vi "Resize Message String & 3-button Dialog Window.vi"(6 "Max Number of Lines":i32, 8 "Error In":errorcluster, 9 "Message":string, 10 "output Controls & Indicators":T1, 11 "VI Refnum":refnum<vi>) -> (0 "Error Out":errorcluster, 3 "VI Refnum out":refnum<vi>)   [LabVIEW 2021, in "GUI.lvlib"]
uses:
  GUI.lvlib
  Error/Error.lvlib
  Buttons/Buttons.lvlib
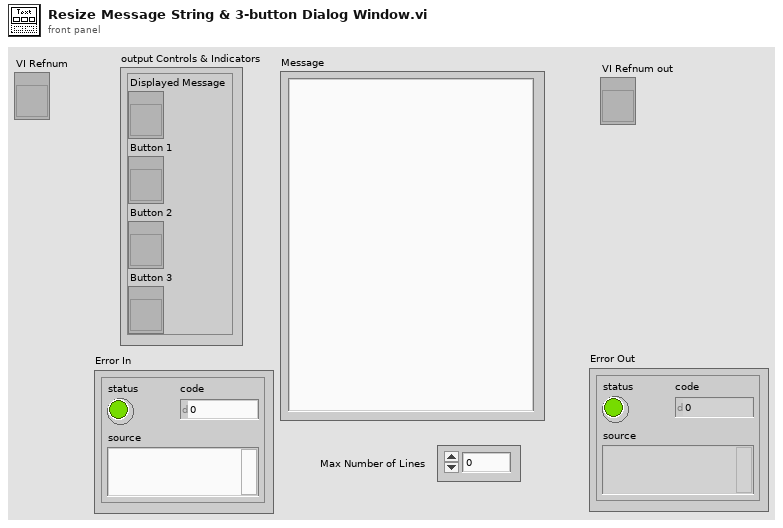
[diagram p1: front panel]
types:
  T1 = cluster{"Displayed Message":refnum<vi>, "Button 1":refnum<vi>, "Button 2":refnum<vi>, "Button 3":refnum<vi>}
  T2 = typedef "LVRectTypeDef.ctl" = cluster{"Left":i16, "Top":i16, "Right":i16, "Bottom":i16}
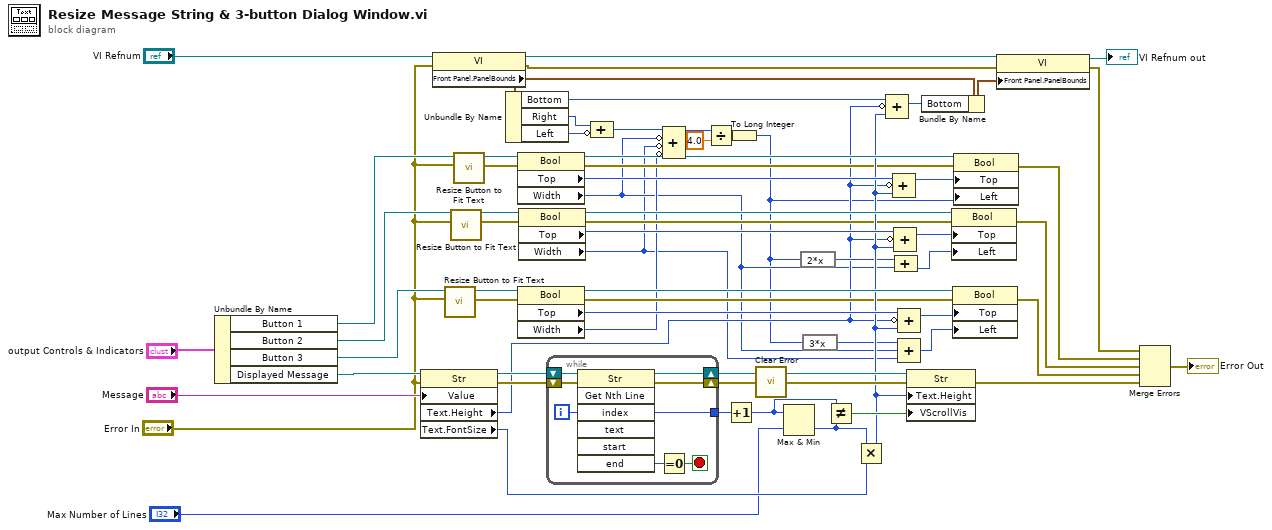
[diagram p0: block diagram]
diagram:
  n1 = Unbundle By Name("output Controls & Indicators") -> ("Button 1"=w13:refnum<vi>, "Button 2"=w21:refnum<vi>, "Button 3"=w41:refnum<vi>, "Displayed Message"=w51:refnum<vi>)
  n2 = property class="Str"(reference=w51, error in="Error In", "Value"="Message") -> (reference out=w65:refnum<vi>, error out=w64:errorcluster, "Text.Height"=w4:u32, "Text.FontSize"=w61:u32)
  n3 = property class="VI"(reference="VI Refnum", error in="Error In") -> (reference out=w47:refnum<vi>, error out=w46:errorcluster, "Front Panel.PanelBounds"=w49:T2)
  n4 = call "Resize Button to Fit Text.vi"("error in (no error)"="Error In", "Boolean in"=w41) -> ("error out"=w22:errorcluster, "Boolean out"=w23:refnum<vi>)  [unwired: 8 in]
  n5 = call "Resize Button to Fit Text.vi"("error in (no error)"="Error In", "Boolean in"=w21) -> ("error out"=w19:errorcluster, "Boolean out"=w20:refnum<vi>)  [unwired: 8 in]
  n6 = call "Resize Button to Fit Text.vi"("error in (no error)"="Error In", "Boolean in"=w13) -> ("error out"=w10:errorcluster, "Boolean out"=w12:refnum<vi>)  [unwired: 8 in]
  n7 = Unbundle By Name(w49) -> ("Bottom"=w50:i16, "Right"=w8:i16, "Left"=w26:i16)
  n8 = property class="Bool"(reference=w12, error in=w10) -> (reference out=w43:refnum<vi>, error out=w32:errorcluster, "Top"=w44:i32, "Width"=w3:u32)
  n9 = property class="Bool"(reference=w23, error in=w22) -> (reference out=w39:refnum<vi>, error out=w30:errorcluster, "Top"=w36:i32, "Width"=w27:u32)
  n10 = property class="Bool"(reference=w20, error in=w19) -> (reference out=w40:refnum<vi>, error out=w31:errorcluster, "Top"=w38:i32, "Width"=w2:u32)
  n11 = while {
    shift-right: [w71] -> w59
    shift-left: w64 -> [w72]
    shift-right: [w70] -> w60
    shift-left: w65 -> [w73]
    tunnel: [w68] -> w62
    i -> [w68]
    stop <- w67 stop-if-true
    n12 = invoke class="Str" method="Get Nth Line"(reference=w73, error in=w72, "index"=w68) -> (reference out=w70:refnum<vi>, error out=w71:errorcluster, "end"=w69:u32)  [unwired: 4 in, 4 out]
    n13 = Equal To 0?(x=w69) -> (x = 0?=w67:bool)
  }
  n14 = Compound Arithmetic op=ADD(w8, invert w26) -> (w25:i16)
  n15 = Compound Arithmetic op=ADD(w25, invert w3, invert w2, invert w27) -> (w29:u32)
  n16 = Divide(x=w29, y=4.0) -> (x/y=w6:dbl)
  n17 = Increment(x=w62) -> (x+1=w55:i32)
  n18 = To Long Integer(number=w6) -> (32bit integer=w1:i32)
  n19 = call "Clear Error.vi"("Error In"=w59) -> ("no Error Out"=w57:errorcluster)  [unwired: 8 in]
  n20 = Max & Min(x=w55, y="Max Number of Lines") -> (min(x,y)=w56:i32)  [unwired: 1 out]
  n21 = expression code="2*x"(w1) -> (w7:i32)
  n22 = expression code="3*x"(w1) -> (w5:i32)
  n23 = Not Equal?(x=w55, y=w56) -> (x != y?=w54:bool)
  n24 = Multiply(x=w56, y=w61) -> (x*y=w35:u32)
  n25 = Compound Arithmetic op=ADD(w50, invert w4, w35) -> (w48:u32)
  n26 = Compound Arithmetic op=ADD(w44, invert w4, w35) -> (w42:u32)
  n27 = Compound Arithmetic op=ADD(w38, invert w4, w35) -> (w37:u32)
  n28 = Compound Arithmetic op=ADD(w7, w3) -> (w9:u32)
  n29 = Compound Arithmetic op=ADD(w36, invert w4, w35) -> (w34:u32)
  n30 = Compound Arithmetic op=ADD(w5, w3, w2) -> (w24:u32)
  n31 = property class="Str"(reference=w60, error in=w57, "Text.Height"=w35, "VScrollVis"=w54) -> (error out=w58:errorcluster)  [unwired: 1 out]
  n32 = Bundle By Name(cluster=w49, "Bottom"=w48) -> (w45:T2)
  n33 = property class="Bool"(reference=w40, error in=w31, "Top"=w37, "Left"=w9) -> (error out=w16:errorcluster)  [unwired: 1 out]
  n34 = property class="Bool"(reference=w39, error in=w30, "Top"=w34, "Left"=w24) -> (error out=w17:errorcluster)  [unwired: 1 out]
  n35 = property class="Bool"(reference=w43, error in=w32, "Top"=w42, "Left"=w1) -> (error out=w15:errorcluster)  [unwired: 1 out]
  n36 = property class="VI"(reference=w47, error in=w46, "Front Panel.PanelBounds"=w45) -> (reference out=→"VI Refnum out":refnum<vi>, error out=w14:errorcluster)
  n37 = Merge Errors(w14, w15, w16, w17, w58) -> (→"Error Out":errorcluster)
